vi "Pause Processing.vi"(8 "error in (no error)":errorcluster, 10 "Internal Message Queue":refnum<queue>, 11 "TestProcessor in":refnum<class "TestProcessor.lvclass">) -> (0 "error out":errorcluster, 3 "TestProcessor out":refnum<class "TestProcessor.lvclass">)   [LabVIEW 2023, in "HAF.lvlib" / "TestProcessor.lvclass"]
doc: "Clear the Internal queue and wait for a Resume message to appear. The queue is reset as Pause messages are raised at the front of the queue (high priority) and no messages originally in the queue should be processed.\n\nProcessing only pauses after the current run through of Command Directors completes."
uses:
  TestProcessor.lvclass
  TestProcessor.lvclass/TestProcessor.ctl
  Message.ctl
  HAF.lvlib
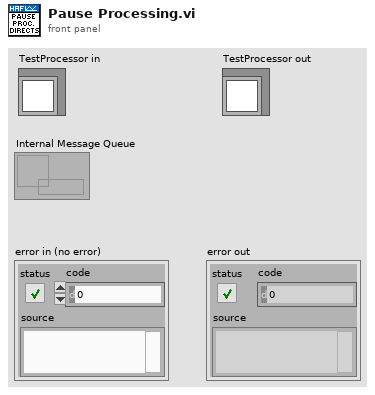
[diagram p1: front panel]
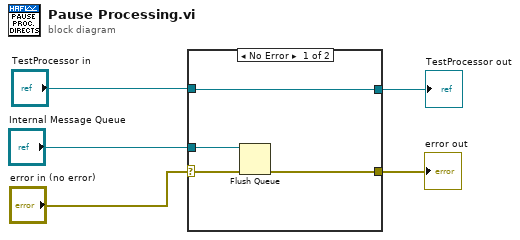
[diagram p0: block diagram]
diagram:
  n1 = case shown="No Error" "error in (no error)" {
    selector: "error in (no error)" -> [w7 w10]
    tunnel: [w9 w10] -> w5
    tunnel: "Internal Message Queue" -> [w8 _]
    tunnel: "TestProcessor in" -> [w6 w11]
    tunnel: [w6 w11] -> w1
    frame No Error {
      n2 = Flush Queue(queue=w8, error in (no error)=w7) -> (error out=w9:errorcluster)  [unwired: 2 out]
    }
    frame Error {
    }
  }
  "error out" <- w5
  "TestProcessor out" <- w1
